vi "Parse-attribute.vi"(8 "error in (no error)":errorcluster, 10 "String in":string, 11 "MarkSpeed in":refnum<class "MarkSpeed.lvclass">) -> (0 "error out":errorcluster, 1 "Valid attribute?":bool, 2 "Remaining string":string, 3 "MarkSpeed out":refnum<class "MarkSpeed.lvclass">)   [LabVIEW 2013, in "MaterialCharacterization.lvlib" / "MarkSpeed.lvclass"]
uses:
  MarkSpeed.lvclass
  Attributes.ctl
  Attribute-ID.ctl
  Attribute-XML.lvclass/Attribute-XML.ctl
  ID.lvclass/ID.ctl
  Speed/Speed.lvclass/Speed.ctl
  Write Attribute.vi
  Write ID-attribute.vi
  Speed/Write Speed.vi
  Speed/Write Update period.vi
  Speed/Write Bits per period.vi
  Speed/Write Components.vi
  Attribute-XML.lvclass
  ID.lvclass
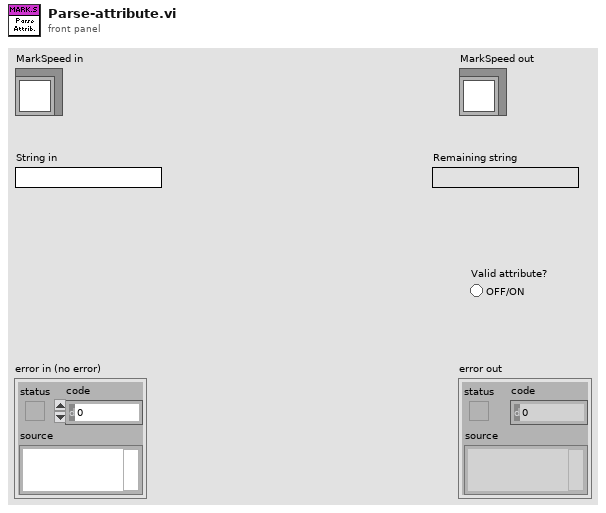
[diagram p1: front panel]
types:
  T1 = typedef "MaterialCharacterization.lvlib/ID.lvclass/Attribute-ID.ctl" = enum16{"FieldOffset", "TransformEnable", "Transform", "Units", "XYCalFactor", "EnableLaser", "JumpDelay", "MarkDelay", "PolyDelay", "LaserOnDelay", "LaserOffDelay", "JumpSpeed", "MarkSpeed", "LaserPowerDelay", "LaserEnableDelay", "LaserPower", "Offset"}
  T2 = typedef "MaterialCharacterization.lvlib/Attribute-XML.lvclass/Attributes.ctl" = enum16{"id"}
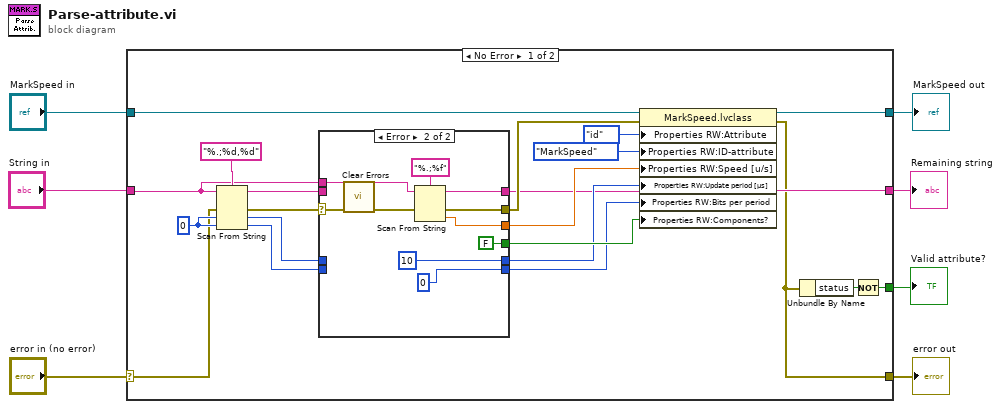
[diagram p0: block diagram]
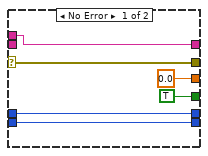
[diagram p2: hidden frame]
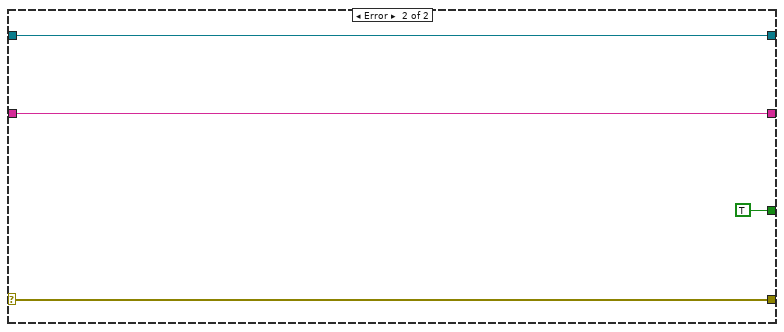
[diagram p3: hidden frame]
diagram:
  n1 = case shown="No Error" "error in (no error)" {
    selector: "error in (no error)" -> [w12 w48]
    tunnel: [w8 w48] -> w6
    tunnel: [w13 w47] -> w4
    tunnel: "MarkSpeed in" -> [w14 w47]
    tunnel: "String in" -> [w11 w46]
    tunnel: [w10 w46] -> w2
    tunnel: [w9 TRUE] -> w1
    frame No Error {
      w24 = u16 0 ("default value 2")
      n2 = Scan From String(format string="%.;%d,%d", input string=w11, error in=w12, default 1=w24, default 2=w24) -> (remaining string=w20:string, error out=w23:errorcluster, output 1=w22:u16, output 2=w21:u16)  [unwired: 1 in, 1 out]
      n3 = case shown="Error" w23 {
        selector: w23 -> [w30 w43]
        tunnel: w22 -> [w34 _]
        tunnel: w21 -> [w33 _]
        tunnel: w11 -> [w29 w42]
        tunnel: w20 -> [_ _]
        tunnel: [w30 w41] -> w19
        tunnel: [0.0 w40] -> w18
        tunnel: [TRUE FALSE] -> w17
        tunnel: [w29 w38] -> w10
        tunnel: [w34 u16 10 ("default value 2")] -> w16
        tunnel: [w33 u16 0 ("default value 2")] -> w15
        frame No Error {
        }
        frame Error {
          n4 = call <vilib>:"Clear Errors.vi"("error in (no error)"=w43) -> ("error out"=w37:errorcluster)  [unwired: 6 in]
          n5 = Scan From String(format string="%.;%f", input string=w42, error in=w37) -> (remaining string=w38:string, error out=w41:errorcluster, output 1=w40:dbl)  [unwired: 2 in, 1 out]
        }
      }
      n6 = property class="MarkSpeed.lvclass"(reference=w14, error in=w19, "Properties RW:Attribute"=Attributes."id" ("Attribute"), "Properties RW:ID-attribute"=Attribute-ID."MarkSpeed" ("ID-attribute"), "Properties RW:Speed [u/s]"=w18, "Properties RW:Update period [µs]"=w16, "Properties RW:Bits per period"=w15, "Properties RW:Components?"=w17) -> (reference out=w13:refnum<class "MarkSpeed.lvclass">, error out=w8:errorcluster)
      n7 = Unbundle By Name(w8) -> ("status"=w27:bool)
      n8 = Not(x=w27) -> (.not. x?=w9:bool)
    }
    frame Error {
    }
  }
  "error out" <- w6
  "MarkSpeed out" <- w4
  "Remaining string" <- w2
  "Valid attribute?" <- w1
